vi "CreateBankChannelsNode.vi"(7 "DOM Document":refnum<k20>, 8 "Error In":errorcluster, 11 "Channel Names":string[](array[string])) -> (0 "Error Out":errorcluster, 3 "Channel Node":refnum<k20>)   [LabVIEW 2012]
uses:
  libs/LV-Utilities/LV-Utilities.lvlib
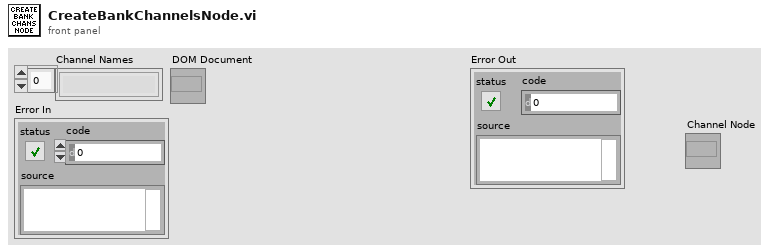
[diagram p1: front panel]
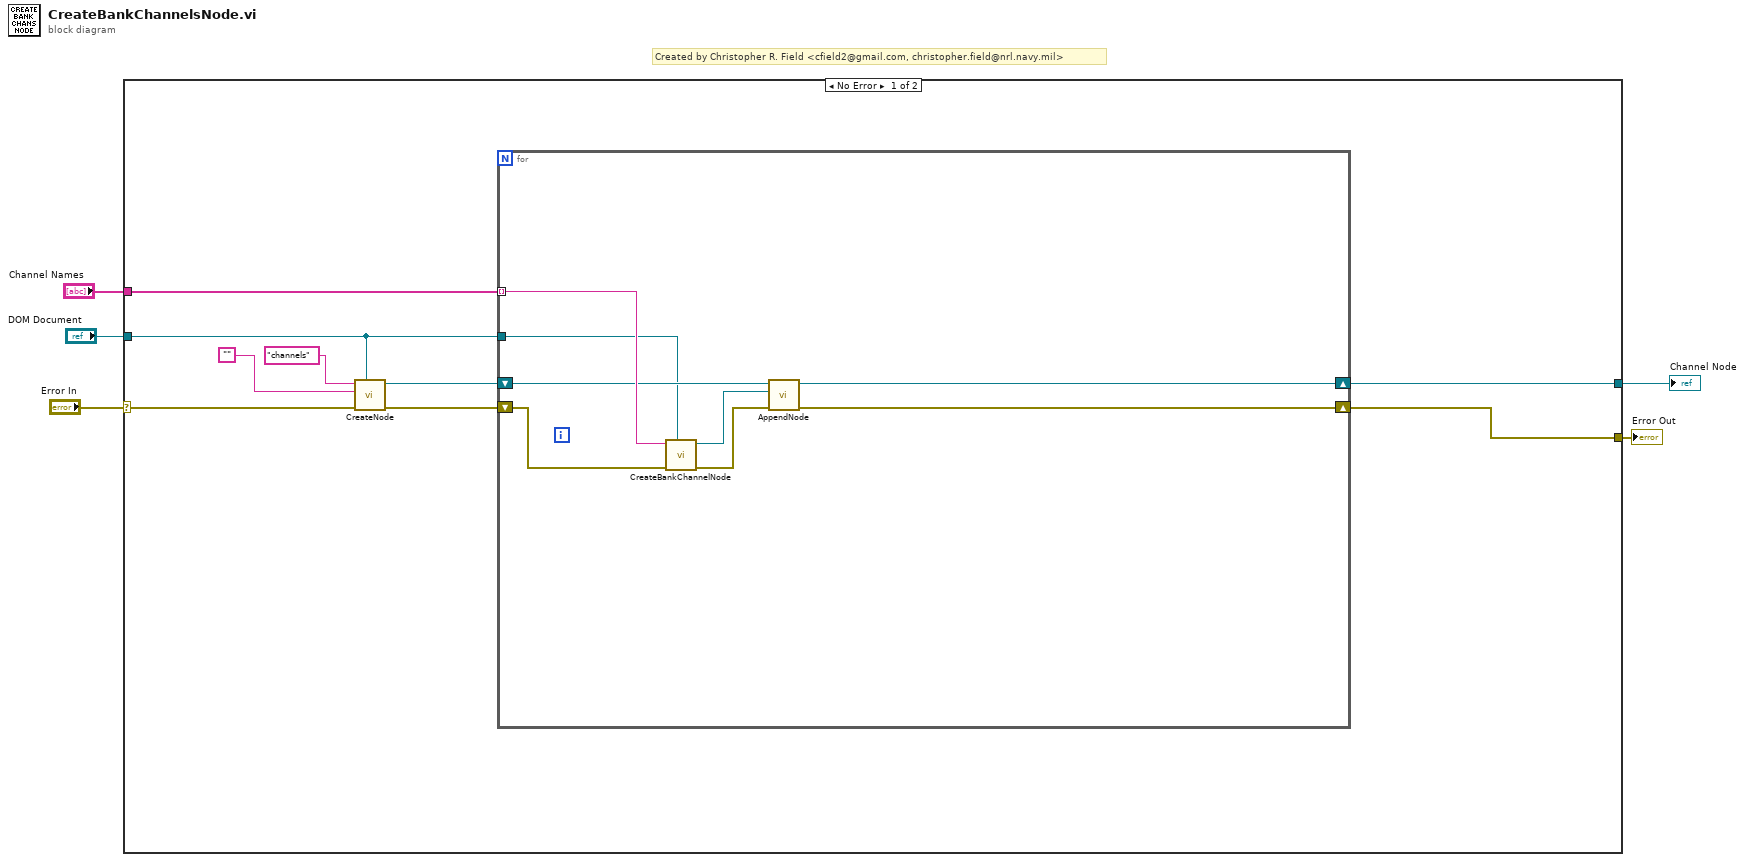
[diagram p0: block diagram]
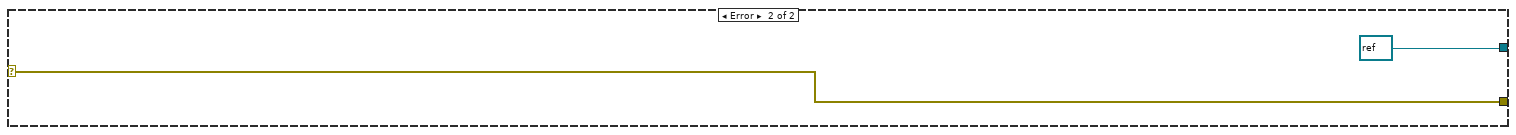
[diagram p2: hidden frame]
diagram:
  # "Created by Christopher R. Field <cfield2@gmail.com, christopher.field@nrl.navy.mil>"
  n1 = case shown="No Error" "Error In" {
    selector: "Error In" -> [w13 w24]
    tunnel: "Channel Names" -> [w14 _]
    tunnel: "DOM Document" -> [w8 _]
    tunnel: [w7 refnum<k20> refnum ("Channel Node 2")] -> w1
    tunnel: [w6 w24] -> w2
    frame No Error {
      n2 = call "CreateNode.vi"("DOM Document"=w8, "Error In"=w13, "Text"="", "Tag Name"="channels") -> ("Error out"=w12:errorcluster, "Node"=w9:refnum<k20>)  [unwired: 6 in]
      n3 = for {
        tunnel: w14 -> [w22] mode=indexing
        shift-right: [w16] -> w6
        shift-left: w12 -> [w21]
        shift-right: [w17] -> w7
        shift-left: w9 -> [w19]
        tunnel: w8 -> [w15]
        n4 = call "CreateBankChannelNode.vi"("DOM Document"=w15, "Error In"=w21, "Channel Name"=w22) -> ("Error Out"=w20:errorcluster, "Bank Channel Node"=w18:refnum<k20>)  [unwired: 7 in]
        n5 = call "AppendNode.vi"("Error In"=w20, "Child Node"=w18, "Parent Node In"=w19) -> ("Error Out"=w16:errorcluster, "Parent Node Out"=w17:refnum<k20>)  [unwired: 7 in]
      }
    }
    frame Error {
    }
  }
  "Error Out" <- w2
  "Channel Node" <- w1
